vi "Convert rpm to radians per sec.vi"(11 "motor speed (rpm)":dbl) -> (3 "speed rps":dbl[unit])   [LabVIEW 2019]
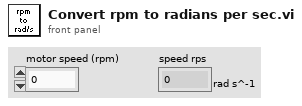
[diagram p1: front panel]
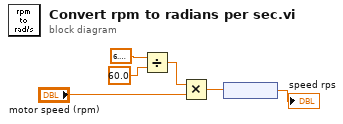
[diagram p0: block diagram]
diagram:
  n1 = Divide(x=6.283185307179586, y=60.0) -> (x/y=w1:dbl)
  n2 = Multiply(x=w1, y="motor speed (rpm)") -> (x*y=w5:dbl)
  n3 = node(w5) -> (→"speed rps":dbl[unit])
